vi "HandleModuleError.vi"(8 "ErrorIn":errorcluster[](array[cluster])) -> (0 "ErrorOut":errorcluster[](array[cluster]))   [LabVIEW 2018]
uses:
  Test.lvclass
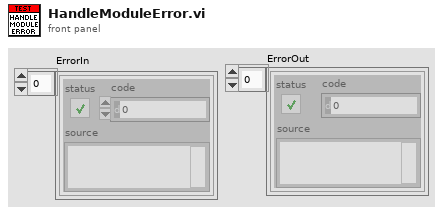
[diagram p1: front panel]
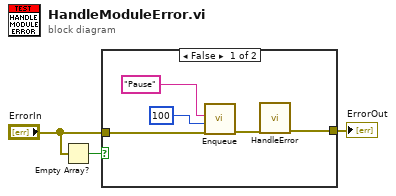
[diagram p0: block diagram]
diagram:
  n1 = Empty Array?(array="ErrorIn") -> (empty?=w2:bool)
  n2 = case shown="False" w2 {
    tunnel: "ErrorIn" -> [w8 w9]
    tunnel: [w4 w9] -> w1
    frame False {
      n3 = call "Enqueue.vi"("ErrorArray"=w8, "Data"=u32 100 ("milliseconds to wait"), "Message"="Pause") -> ("ErrorArray"=w5:errorcluster[])  [unwired: 8 in]
      n4 = call "HandleError.vi"("ErrorArray"=w5) -> ("ErrorArray"=w4:errorcluster[])  [unwired: 8 in, 2 out]
    }
    frame True {
    }
  }
  "ErrorOut" <- w1
